vi "Sinusoids.vi"() -> ()   [LabVIEW 2012]
uses:
  <vilib>/picture/picture.llb/Draw 8-Bit Pixmap.vi
  <vilib>/imath/engines/lvmath2/RunTimeEngine/ErrorHandling/NIMS_Finalize Error.vi
  <vilib>/imath/engines/lvmath2/RunTimeEngine/Managers/WorkSpace/UID Generator.vi
  <vilib>/imath/engines/lvmath2/RunTimeEngine/Managers/SymbolTable/Clear UID.vi
  <vilib>/imath/engines/lvmath2/RunTimeEngine/NodeEndStatement/NIMS_NodeEndStatement_Output.vi
  <instcachedir>/0/NIMS_NodeEndStatement_Output_53EC0D466D134D7ABD903AC30B43404B.lvgen/NIMS_NodeEndStatement_Output_53EC0D466D134D7ABD903AC30B43404B_009.vi
  <vilib>/imath/engines/lvmath2/RunTimeEngine/RunTimeType/NIMS_RunTimeType_From StrictType (excl LVString).vi
  <instcachedir>/0/NIMS_RunTimeType_From StrictType (excl LVString)_27CFCE38286AFF43ABD3E48A72A09368.lvgen/NIMS_RunTimeType_From StrictType (excl LVString)_27CFCE38286AFF43ABD3E48A72A09368_000.vi
  <vilib>/imath/engines/lvmath2/RunTimeEngine/LocalVariableDefStatement/MC_LocalVariableDefStatement_Display.vi
  <vilib>/imath/engines/lvmath2/RunTimeEngine/RangeToken/NIMS_Range_R2 - Integer.vi
  <instcachedir>/0/NIMS_Range_R2 - Integer_AAD493E2D93985418B87E485D4769DC2.lvgen/NIMS_Range_R2 - Integer_AAD493E2D93985418B87E485D4769DC2_000.vi
  <vilib>/imath/engines/lvmath2/RunTimeEngine/CommandStatement/MC_CommandStatement_break.vi
  <vilib>/imath/engines/lvmath2/RunTimeEngine/ReplaceToken/NIMS_Replace - Check Linear.vi
  <instcachedir>/0/NIMS_Replace - Check Linear_6C45E163336FD74D99F8103F7D880A40.lvgen/NIMS_Replace - Check Linear_6C45E163336FD74D99F8103F7D880A40_008.vi
  <vilib>/imath/engines/lvmath2/RunTimeEngine/BuiltInFunctions/uint8/NIMS_uint8(real).vi
  <instcachedir>/0/NIMS_uint8(real)_CAA419FBB1354DA296C59E18C46DECF0.lvgen/NIMS_uint8(real)_CAA419FBB1354DA296C59E18C46DECF0_000.vi
  <vilib>/imath/engines/lvmath2/RunTimeEngine/ReplaceToken/NIMS_Replace - Size Check _(_)=S.vi
  <instcachedir>/0/NIMS_Replace - Size Check _(_)=S_F1238981F30EF84688488EE257E7CC3F.lvgen/NIMS_Replace - Size Check _(_)=S_F1238981F30EF84688488EE257E7CC3F_006.vi
  <vilib>/imath/engines/lvmath2/RunTimeEngine/ReplaceToken/NIMS_Replace - V(S)=S.vi
  <instcachedir>/0/NIMS_Replace - V(S)=S_6D54BA4C4C35E94EBB08DF4C480EEF51.lvgen/NIMS_Replace - V(S)=S_6D54BA4C4C35E94EBB08DF4C480EEF51_003.vi
  <vilib>/imathl/engines/lvmath/Functions/Error Handling/Create Error.vi
  <vilib>/imath/engines/lvmath2/RunTimeEngine/BuiltInFunctions/repeatmx/NIMS_repeatmx(GM, I32, I32).vi
  <instcachedir>/0/NIMS_repeatmx(GM, I32, I32)_6EF7819D61DDB34FA8EBD413A05A61A3.lvgen/NIMS_repeatmx(GM, I32, I32)_6EF7819D61DDB34FA8EBD413A05A61A3_004.vi
  <vilib>/imath/engines/lvmath2/RunTimeEngine/Managers/SymbolTable/NIMS_WorkSpace.lvlib
panel:
  in  "Variable Gradient":dbl(slide) scale=0.0..10.0
  out "Horizontal Variable Gradient 2":picture
  out "Horizontal Gradient":picture
  out "Vertical Gradient":picture
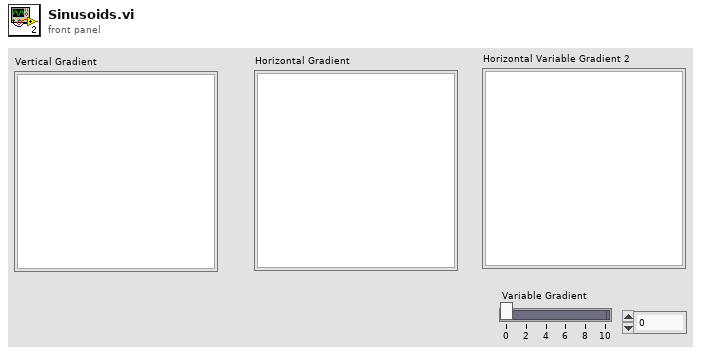
[diagram p1: front panel]
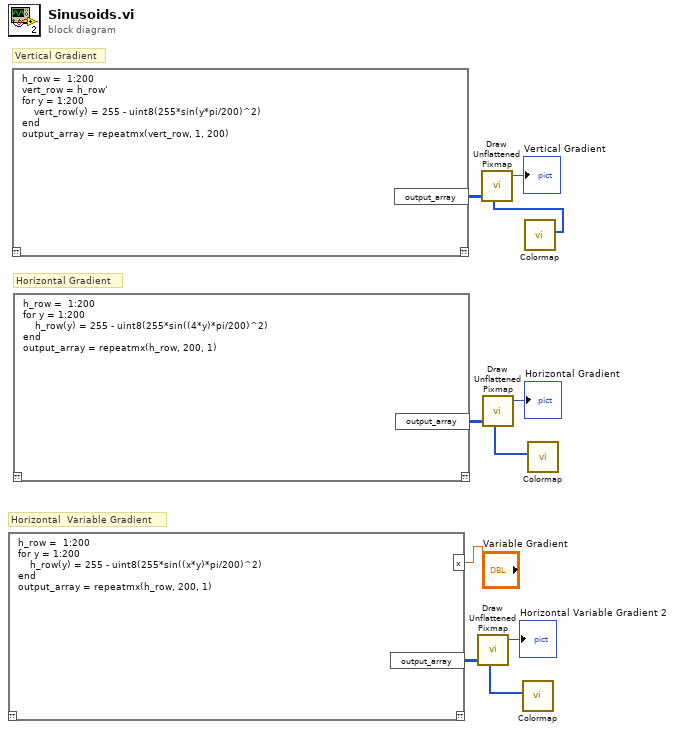
[diagram p0: block diagram]
diagram:
  # "Horizontal  Variable Gradient"
  # "Vertical Gradient"
  # "Horizontal Gradient"
  n1 = mathscript code="h_row =  1:200\nfor y = 1:200\n    h_row(y) = 255 - uint8(255*sin((x*y)*pi/200)^2)\nend\noutput_array = repeatmx(h_row, 200, 1)"("x"="Variable Gradient") -> ("output_array"=w2:i32[][])  [unwired: 1 in, 1 out]
  n2 = mathscript code="h_row =  1:200\nvert_row = h_row'\nfor y = 1:200\n    vert_row(y) = 255 - uint8(255*sin(y*pi/200)^2)\nend\noutput_array = repeatmx(vert_row, 1, 200)"() -> ("output_array"=w8:i32[][])  [unwired: 1 in, 1 out]
  n3 = mathscript code="h_row =  1:200\nfor y = 1:200\n    h_row(y) = 255 - uint8(255*sin((4*y)*pi/200)^2)\nend\noutput_array = repeatmx(h_row, 200, 1)"() -> ("output_array"=w5:i32[][])  [unwired: 1 in, 1 out]
  n4 = call "Colormap.vi"() -> ("Array"=w4:u32[])  [unwired: 11 in]
  n5 = call-poly <vilib>:"Draw Unflattened Pixmap.vi"("data"=w2, "color table"=w4) -> ("new picture"=→"Horizontal Variable Gradient 2":picture)  [unwired: 7 in]
  n6 = call "Colormap.vi"() -> ("Array"=w10:u32[])  [unwired: 11 in]
  n7 = call-poly <vilib>:"Draw Unflattened Pixmap.vi"("data"=w8, "color table"=w10) -> ("new picture"=→"Vertical Gradient":picture)  [unwired: 7 in]
  n8 = call "Colormap.vi"() -> ("Array"=w7:u32[])  [unwired: 11 in]
  n9 = call-poly <vilib>:"Draw Unflattened Pixmap.vi"("data"=w5, "color table"=w7) -> ("new picture"=→"Horizontal Gradient":picture)  [unwired: 7 in]
